vi "Start key.vi"(8 "error in":errorcluster) -> (0 "error out":errorcluster, 3 "Clinder Up":bool)   [LabVIEW 2009]
uses:
  Digit IO control.ctl
  <vilib>/DAQmx/read.llb/DAQmx Read (Digital Bool 1Line 1Point).vi
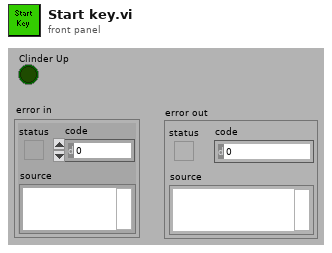
[diagram p1: front panel]
types:
  T1 = typedef "Digit IO control.ctl" = enum16{"Pull X1_4 Low", "Disconnect Pull X1_4 Low", "Down Cylinder", "Disconnect Down Cylinder", "Load X1_1_5", "Disconnect Load X1_1_5", "Measu X1_1_5", "Disconnect Measu X1_1_5", "Measu Z1_1_5", "Disconnect Measu Z1_1_5", "Power X1_1", "Disconnect Power X1_1", "RS232 Power", "Disconnect RS232 Power", "Card Cylinder", "Disconnect Card Cylinder", "Fail LED", "Disconnect Fail LED", "LCA Power", "Disconnect LCA Power", "BeyondCylinderDowndigit", "Disconnect BeyondCylinderDowendigit", "Frequency", "Disconnect Frequency", "Measu Current", "Disconnect Measu Current", "Measu current_1", "Disconnect Measu current_1", "Digit ALL", "Disconnect Digit ALL", "PASS LED", "Disconnect PASS LED", "Load Z1_1_3", "Disconnect Load Z1_1_3", "RS232 Connect", "Disconnect RS232 Connect", "Power Z1_7", "Disconnect Power Z1_7", "Pull Z_1_5  low", "Disconnect Pull Z_1_5  low", "Connect LCA_1", "Disconnect LCA_1", "short LCA", "Disconnect short LCA", "PT100", "Disconnect PT100", "NO connect", "Disconnect NO connect"}
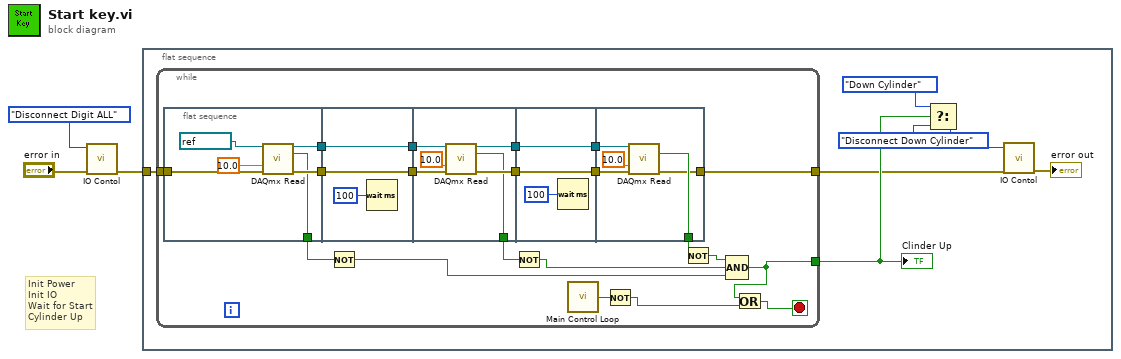
[diagram p0: block diagram]
diagram:
  # "Init Power\nInit IO\nWait for Start\nCylinder Up"
  n1 = call "IO Contol.vi"("error in"="error in", "IO Operation"=Digit_IO_control."Disconnect Digit ALL") -> ("error out"=w3:errorcluster)  [unwired: 9 out]
  n2 = flat-sequence {
    tunnel: w3 -> [w7]
    frame #0 {
      n3 = while {
        tunnel: [w13] -> w8
        tunnel: [w16] -> w5
        tunnel: w7 -> [w15]
        stop <- w11 stop-if-true
        n4 = flat-sequence {
          tunnel: [w34] -> w29
          tunnel: [w33] -> w25
          tunnel: [w32] -> w22
          tunnel: w15 -> [w31]
          tunnel: [w38] -> w30
          tunnel: w29 -> [w38]
          tunnel: [w37] -> w26
          tunnel: w25 -> [w37]
          tunnel: w30 -> [w45]
          tunnel: [w44] -> w27
          tunnel: w26 -> [w43]
          tunnel: [w42] -> w23
          tunnel: [w40] -> w21
          tunnel: [w47] -> w28
          tunnel: w27 -> [w47]
          tunnel: [w46] -> w24
          tunnel: w23 -> [w46]
          tunnel: w28 -> [w53]
          tunnel: w24 -> [w52]
          tunnel: [w50] -> w20
          tunnel: [w49] -> w16
          frame #0 {
            n5 = call-poly <vilib>:"DAQmx Read.vi"("task/channels in"=refnum<k21> "Start" ("DAQmx Global Channel"), "timeout"=10.0, "error in"=w31) -> ("task out"=w33:refnum<k21>, "data"=w32:bool, "error out"=w34:errorcluster)  [unwired: 10 out]
          }
          frame #1 {
            n6 = Wait (ms)(milliseconds to wait=u32 100) -> ()  [unwired: 1 out]
          }
          frame #2 {
            n7 = call-poly <vilib>:"DAQmx Read.vi"("task/channels in"=w43, "timeout"=10.0, "error in"=w45) -> ("task out"=w42:refnum<k21>, "data"=w40:bool, "error out"=w44:errorcluster)  [unwired: 10 out]
          }
          frame #3 {
            n8 = Wait (ms)(milliseconds to wait=u32 100) -> ()  [unwired: 1 out]
          }
          frame #4 {
            n9 = call-poly <vilib>:"DAQmx Read.vi"("task/channels in"=w52, "timeout"=10.0, "error in"=w53) -> ("data"=w50:bool, "error out"=w49:errorcluster)  [unwired: 11 out]
          }
        }
        n10 = Not(x=w22) -> (.not. x?=w18:bool)
        n11 = Not(x=w21) -> (.not. x?=w19:bool)
        n12 = call "Main Control Loop.vi"() -> ("Loop Out"=w14:bool)  [unwired: 1 in, 4 out]
        n13 = Not(x=w14) -> (.not. x?=w12:bool)
        n14 = Not(x=w20) -> (.not. x?=w17:bool)
        n15 = Compound Arithmetic op=AND(w17, w19, w18) -> (w13:bool)
        n16 = Or(x=w13, y=w12) -> (x .or. y?=w11:bool)
      }
      "Clinder Up" <- w8
      n17 = Select(t=Digit_IO_control."Down Cylinder" ("Enum"), s=w8, f=Digit_IO_control."Disconnect Down Cylinder" ("Enum")) -> (s? t:f=w6:T1)
      n18 = call "IO Contol.vi"("error in"=w5, "IO Operation"=w6) -> ("error out"=→"error out":errorcluster)  [unwired: 9 out]
    }
  }
